vi "Page_Preview_Update_Tree_Icons.vi"(7 "Preview Tree":refnum<vi>, 8 "error in (no error)":errorcluster, 11 "AB_Deploy_EXE in":refnum<class "AB_Deploy_EXE.lvclass">) -> (0 "error out":errorcluster, 3 "AB_Deploy_EXE out":refnum<class "AB_Deploy_EXE.lvclass">)   [LabVIEW 2020, in "AB_Deploy_EXE.lvclass"]
uses:
  <vilib>/AppBuilder/AB_Classes/DeployableEXE/AB_Deploy_EXE.lvclass
  <vilib>/AppBuilder/AB_Classes/DeployableEXE/AB_Deploy_EXE.lvclass/AB_Deploy_EXE.ctl
  <vilib>/AppBuilder/AB_Classes/Build/AB_Build.lvclass
  <vilib>/AppBuilder/AB_Classes/Destination/AB_Destination.lvclass
  <vilib>/AppBuilder/AB_Classes/EXE/AB_EXE.lvclass
  <vilib>/AppBuilder/AB_Classes/TargetFile/AB_Targetfile.lvclass
  e:/builds/penguin/labview/branches/2020/dev/dist/vi.lib/AppBuilder/AB_Classes/EXE/AB_EXE.lvclass
  e:/builds/penguin/labview/branches/2020/dev/dist/vi.lib/AppBuilder/AB_Classes/Application/AB_Application.lvclass
  e:/builds/penguin/labview/branches/2020/dev/dist/vi.lib/AppBuilder/AB_Classes/TargetFile/AB_Targetfile.lvclass
  e:/builds/penguin/labview/branches/2020/dev/dist/vi.lib/AppBuilder/AB_Classes/Build/AB_Build.lvclass
  e:/builds/penguin/labview/branches/2020/dev/dist/vi.lib/AppBuilder/AB_Classes/DeployableEXE/AB_Deploy_EXE.lvclass
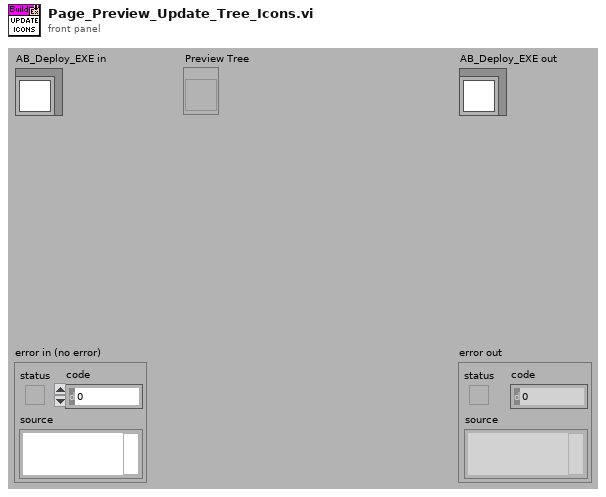
[diagram p1: front panel]
types:
  T1 = typedef "AB_Build.ctl" = cluster{"buildSpecName":string, "buildSpecDescription":string, "destinations":refnum<class "AB_Destination.lvclass">[], "exclusionOption":T2, "defaultLanguage":string, "supportedLanguages":string[], "excludedDirectories":path[], "buildContext":refnum<vi>, "buildObject":T3, "preview":bool, "programatic":bool, "progressBarEvents":T4, "userLog_Path":path, "preActionID":string, "preAction_Path":path, "postActionID":string, "postAction_Path":path, "eng_checkForBrokenVIs?":bool, "eng_verboseLinkerErrors?":bool, "localDest_Path":path, "targetDest_Path":path, "removeVIObject":u16, "cache":refnum<class "PreviewCache.lvclass">, "use cache":bool, "previewCache_ID":string, "buildCache_ID":string, "eng_TempLocalDest_Path":path, "eng_collectDependencies?":bool, "versionInfo":cluster{"buildVersion":cluster{"major":u16, "minor":u16, "patch":u16, "build":u16}, "autoIncrement":bool}, "eng_enableVIChecksums":bool}
  T2 = typedef "AB_Exclusion_Option.ctl" = cluster{"typedefs":bool, "polymorphicVIs":bool, "unusedLibraryItems":bool, "modifyLibraryFile":bool, "edit-timeDependencies":bool, "inlineVIs":bool, "dependent PPLs":bool, "dependent DLLs":bool}
  T3 = typedef "ItemRef.ctl" = u64
  T4 = typedef "provcom_ProgressBar_Events.ctl" = cluster{"newJob":refnum<user-event>, "newItem":refnum<user-event>, "errorMsg":T5, "cancel":refnum<user-event>}
  T5 = typedef "mxLvBuildError.ctl" = refnum<user-event>
  T6 = typedef "AB_Targetfile.ctl" = cluster{"targetfileName":string, "targetfileGUID":string, "enableDebugging":bool, "versionInfo":cluster{"productName":string, "legalCopyright":string, "companyName":string, "internalName":string, "fileDescription":string}, "eng_consolidatedTypeInfo":string, "fastFileFormat":bool, "eng_LEIFBuildData":u32, "versionIndependent":bool}
  T7 = typedef "AB_Destination.ctl" = cluster{"destName":string, "path":path, "libraryName":string, "preserveHierarchy":bool, "eng_inBuild":bool, "eng_libraryReference":refnum<vi>, "eng_restictAddToNewLibrary":bool}
  T8 = typedef "AB_EXE.ctl" = cluster{"cmdLineArgs":bool, "actXServerName":string, "actXServerNameGUID":string, "iconPath":path, "iconItemID":string, "var deploy data":T9}
  T9 = typedef "AB_EXE_SharedVar_Deploy.ctl" = cluster{"deploy at startup":bool, "undeploy on exit":bool, "variable libraries":T10[], "hide deployment dialog":bool}
  T10 = typedef "AB_EXE_SharedVar_LibInfo.ctl" = cluster{"LibraryPath":path, "LibraryItemID":string, "target":string, "deploy":bool}
  T11 = typedef "imagedata.ctl" = cluster{"image type":i32, "image depth":i32, "image":u8[], "mask":u8[], "colors":u32[], "Rectangle":cluster{"left":i16, "top":i16, "right":i16, "bottom":i16}}
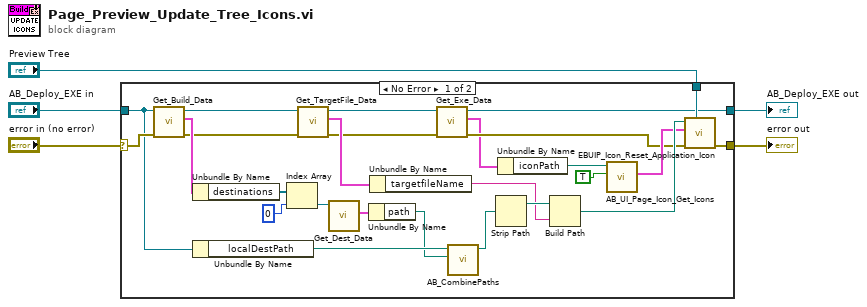
[diagram p0: block diagram]
diagram:
  n1 = case shown="No Error" "error in (no error)" {
    selector: "error in (no error)" -> [w17 w32]
    tunnel: "AB_Deploy_EXE in" -> [w9 w33]
    tunnel: [w13 w33] -> w4
    tunnel: "Preview Tree" -> [w18 _]
    tunnel: [w15 w32] -> w1
    frame No Error {
      n2 = call <vilib>:"Get_Build_Data.vi"("error in (no error)"=w17, "Class in"=w9) -> ("error out"=w16:errorcluster, "data"=w31:T1, "Class out"=w22:refnum<class "AB_Deploy_EXE.lvclass">)  [unwired: 7 in]
      n3 = Unbundle By Name(w31) -> ("destinations"=w30:refnum<class "AB_Destination.lvclass">[])
      n4 = Unbundle By Name(w9) -> ("localDestPath"=w8:path)
      n5 = Index Array(array=w30, index=0) -> (element=w26:refnum<class "AB_Destination.lvclass">)
      n6 = call <vilib>:"Get_TargetFile_Data.vi"("error in (no error)"=w16, "AB_Targetfile in"=w22) -> ("error out"=w12:errorcluster, "data"=w25:T6, "AB_Targetfile out"=w14:refnum<class "AB_Deploy_EXE.lvclass">)  [unwired: 7 in]
      n7 = call <vilib>:"Get_Dest_Data.vi"("Class in"=w26) -> ("destName"=w27:T7)  [unwired: 8 in, 2 out]
      n8 = Unbundle By Name(w27) -> ("path"=w7:path)
      n9 = Unbundle By Name(w25) -> ("targetfileName"=w24:string)
      n10 = call <vilib>:"Get_Exe_Data.vi"("error in (no error)"=w12, "Class in"=w14) -> ("error out"=w11:errorcluster, "data"=w10:T8, "Class out"=w13:refnum<class "AB_Deploy_EXE.lvclass">)  [unwired: 7 in]
      n11 = call <vilib>:"AB_CombinePaths.vi"("target path"=w7, "localDestPath"=w8) -> ("combined path"=w6:path)  [unwired: 9 in]
      n12 = Strip Path(path=w6) -> (stripped path=w28:path)  [unwired: 1 out]
      n13 = Unbundle By Name(w10) -> ("iconPath"=w21:path)
      n14 = Build Path(base path=w28, name or relative path=w24) -> (appended path=w20:path)
      n15 = call <resource>:"AB_UI_Page_Icon_Get_Icons.vi"("preview?"=TRUE, "Icon path"=w21) -> ("preview image data"=w19:T11)  [unwired: 6 in, 3 out]
      n16 = call <resource>:"EBUIP_Icon_Reset_Application_Icon.vi"("Preview Tree"=w18, "error in (no error)"=w11, "Application Icon"=w19, "Application Path"=w20) -> ("error out"=w15:errorcluster)  [unwired: 7 in]
    }
    frame Error {
    }
  }
  "error out" <- w1
  "AB_Deploy_EXE out" <- w4
